vi "GET_PORT_CONN_TYPE.vi"(0 "VNA":refnum<visa-resource-name>, 11 "error in":errorcluster, 12 "Channel":i32, 13 "NumOfPorts":i32=4) -> (4 "VNA Out":refnum<visa-resource-name>, 8 "Conns":string[](array[string]), 15 "error out":errorcluster)   [LabVIEW 2018, in "PNA-X.lvlib"]
uses:
  PNA-X.lvlib
  Instance           1 26Saved   GET_PORT_CONN_TYPE .vi
panel:
  out "CalKit":string[](array[string])
  in  "Calibration Kit":string(combo)="N4691-60004 ECal"
  out "PORT #":i32
  in  "OK Button":bool
  in  "Connector Type":i32(listbox)
  # "Select  'Not used' for Inactive ports."
  # "Select or Enter Cal Kit"
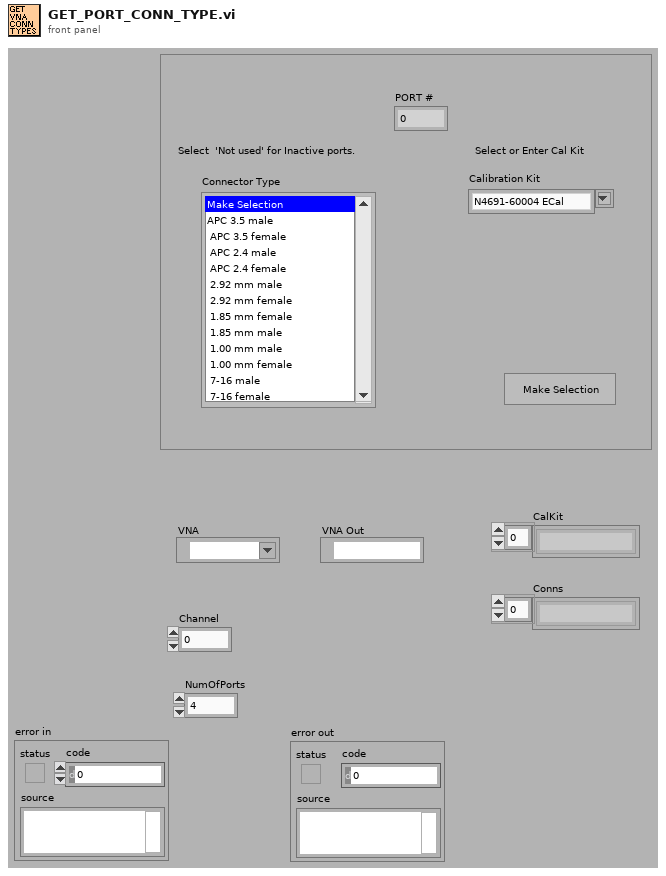
[diagram p1: front panel]
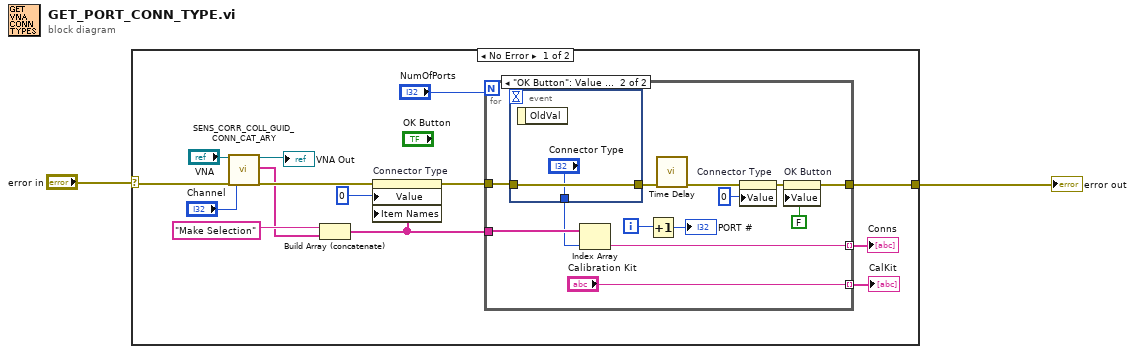
[diagram p0: block diagram]
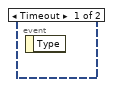
[diagram p2: hidden frame]
diagram:
  n1 = case shown="No Error" "error in" {
    selector: "error in" -> [w11 w32]
    tunnel: [w14 w32] -> w1
    frame No Error {
      n2 = call "SENS_CORR_COLL_GUID_CONN_CAT_ARY.vi"("VNA"="VNA", "error in"=w11, "Channel"="Channel") -> ("VNA Out"=→"VNA Out":refnum<visa-resource-name>, "ConAry"=w8:string[], "error out"=w9:errorcluster)  [unwired: 14 in]
      n3 = Build Array (concatenate)("Make Selection", w8) -> (w13:string[])
      n4 = property on="Connector Type" class="LstBox (strict)"(error in=w9, "Value"=0 ("Connector Type"), "Item Names"=w13) -> (error out=w15:errorcluster)  [unwired: 1 in, 1 out]
      n5 = for {
        N: "NumOfPorts" -> [_]
        tunnel: w15 -> [w29]
        tunnel: [w18] -> w14
        tunnel: w13 -> [w28]
        tunnel: [w27] -> w4 mode=indexing
        tunnel: ["Calibration Kit"] -> w3 mode=indexing
        i -> [w21]
        n6 = event shown="[1] \"OK Button\": Value Change" {
          selector: _ -> [_ _]
          dyn-events: _ -> [_ _]
          timeout: _ -> [_ _]
          tunnel: w29 -> [_ w31]
          tunnel: [_ w31] -> w24
          tunnel: [_ "Connector Type"] -> w25
          event Timeout {
            n7 = event-data() -> ()  [unwired: 1 in, 1 out]
          }
          event "OK Button": Value Change {
            n8 = event-data() -> ()  [unwired: 1 in, 1 out]
          }
        }
        n9 = Index Array(array=w28, index=w25) -> (element=w27:string)
        n10 = Increment(x=w21) -> (x+1=→"PORT #":i32)
        n11 = call "Time Delay"("error in (no error)"=w24) -> ("error out"=w23:errorcluster)  [unwired: 10 in]
        n12 = property on="Connector Type" class="LstBox (strict)"(error in=w23, "Value"=0 ("Connector Type")) -> (error out=w19:errorcluster)  [unwired: 1 in, 1 out]
        n13 = property on="OK Button" class="Bool (strict)"(error in=w19, "Value"=FALSE) -> (error out=w18:errorcluster)  [unwired: 1 in, 1 out]
      }
      "Conns" <- w4
      "CalKit" <- w3
    }
    frame Error {
    }
  }
  "error out" <- w1
